vi "Set System Image (File).vi"(4 "File and Directory Blacklist":string[](array[string]), 5 "Encryption Passphrase":string, 6 "Original System Only (F)":bool, 7 "Restart Automatically (T)":bool=TRUE, 8 "error in (no error)":errorcluster, 9 "Network Settings (preserve primary adapter, apply others)":T1=3 items=["reset all network adapters", "preserve primary, reset others", "preserve all network adapters", "preserve primary, apply others", "apply primary, reset others", "apply primary, preserve others", "apply all network adapters"], 10 "Source File":path, 11 "Session in":refnum<k21>) -> (0 "error out":errorcluster, 3 "Session out":refnum<k21>)   [LabVIEW 2014, in "nisyscfg.lvlib"]
doc: "Replaces the entire contents of the primary hard drive on a specified target system with an image file created with the Create System Image VI."
uses:
  nisyscfg.lvlib
  Network Settings Image.ctl
  NI_Unzip.lvlib
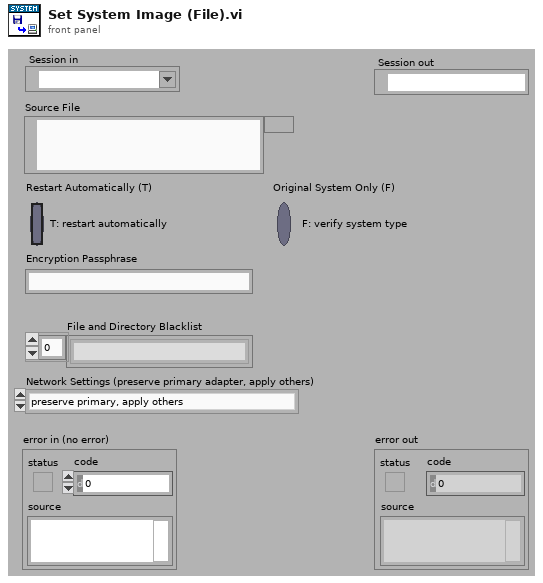
[diagram p1: front panel]
types:
  T1 = typedef "nisyscfg.lvlib/Network Settings Image.ctl" = u32
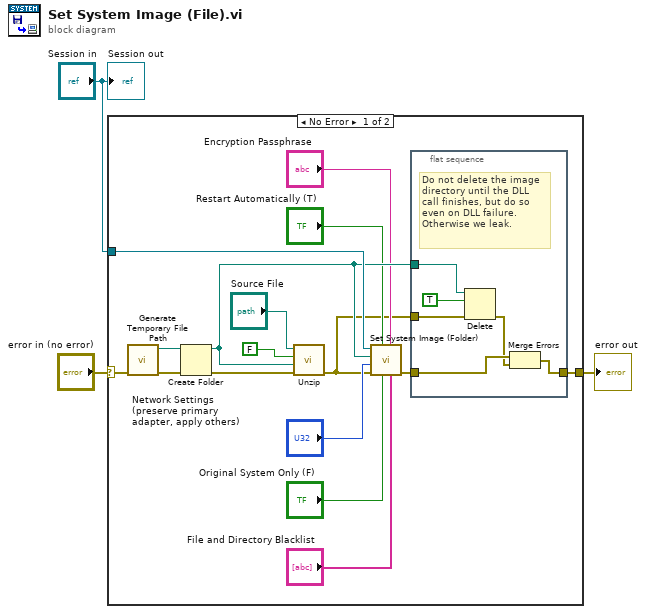
[diagram p0: block diagram]
diagram:
  n1 = case shown="No Error" "error in (no error)" {
    selector: "error in (no error)" -> [w17 w26]
    tunnel: [w4 w26] -> w3
    tunnel: "Session in" -> [w13 _]
    frame No Error {
      n2 = call "Generate Temporary File Path.vi"("error in (no error)"=w17) -> ("error out"=w19:errorcluster, "Unique Temporary File Path"=w18:path)  [unwired: 9 in]
      n3 = Create Folder(path (use dialog)=w18, error in=w19) -> (created path=w12:path, error out=w14:errorcluster)  [unwired: 1 in, 1 out]
      n4 = call "Unzip.vi"("error in (no error)"=w14, "Target directory (same as Zip file if empty)"=w12, "Preview only?"=FALSE, "Zip file"="Source File") -> ("error out"=w6:errorcluster)  [unwired: 7 out]
      n5 = call "Set System Image (Folder).vi"("File and Directory Blacklist"="File and Directory Blacklist", "Encryption Passphrase"="Encryption Passphrase", "Original System Only (F)"="Original System Only (F)", "Restart Automatically (T)"="Restart Automatically (T)", "error in (no error)"=w6, "Network Settings (preserve primary adapter, apply others)"="Network Settings (preserve primary adapter, apply others)", "Source Folder"=w12, "Session in"=w13) -> ("error out"=w5:errorcluster)  [unwired: 2 in, 1 out]
      n6 = flat-sequence {
        tunnel: w12 -> [w24]
        tunnel: w6 -> [w23]
        tunnel: w5 -> [w21]
        tunnel: [w22] -> w4
        frame #0 {
          # "Do not delete the image\ndirectory until the DLL\ncall finishes, but do so\neven on DLL failure.\nOtherwise we leak."
          n7 = Delete(path (use dialog)=w24, entire hierarchy (F)=TRUE, error in=w23) -> (error out=w20:errorcluster)  [unwired: 2 in, 2 out]
          n8 = Merge Errors(w21, w20) -> (w22:errorcluster)
        }
      }
    }
    frame Error {
    }
  }
  "error out" <- w3
  "Session out" <- "Session in"
